vi "IPC-MQTT-Q driver.vi"(6 "Q Options":T2=enum."En Q N", 8 "error in (no error)":errorcluster, 9 "Message Data":variant, 10 "En Q":T1[](array[typedef]), 11 "Message":string) -> (0 "error out":errorcluster, 2 "Data":variant, 3 "State":string)   [LabVIEW 2020]
uses:
  Controls/IPC-MQTT-Q driver-Q Options.ctl
  Controls/IPC-MQTT-Q driver-En Q Element.ctl
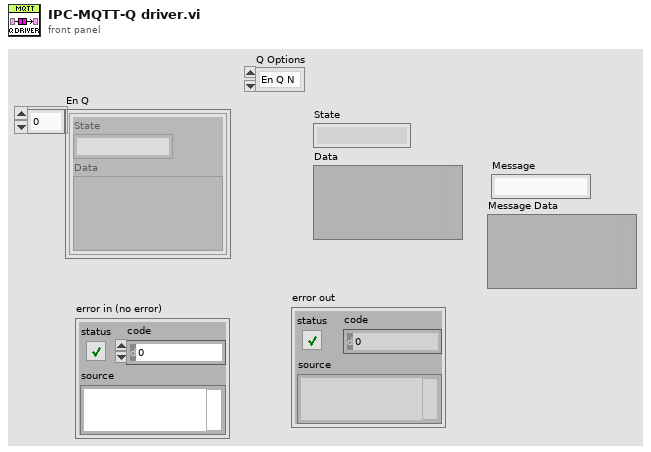
[diagram p1: front panel]
types:
  T1 = typedef "IPC-MQTT-Q driver-En Q Element.ctl" = cluster{"State":string, "Data":variant}
  T2 = typedef "IPC-MQTT-Q driver-Q Options.ctl" = enum16{"En Q", "En Q N", "De Q", "Init", "En Q N Stack", "Flush", "Close"}
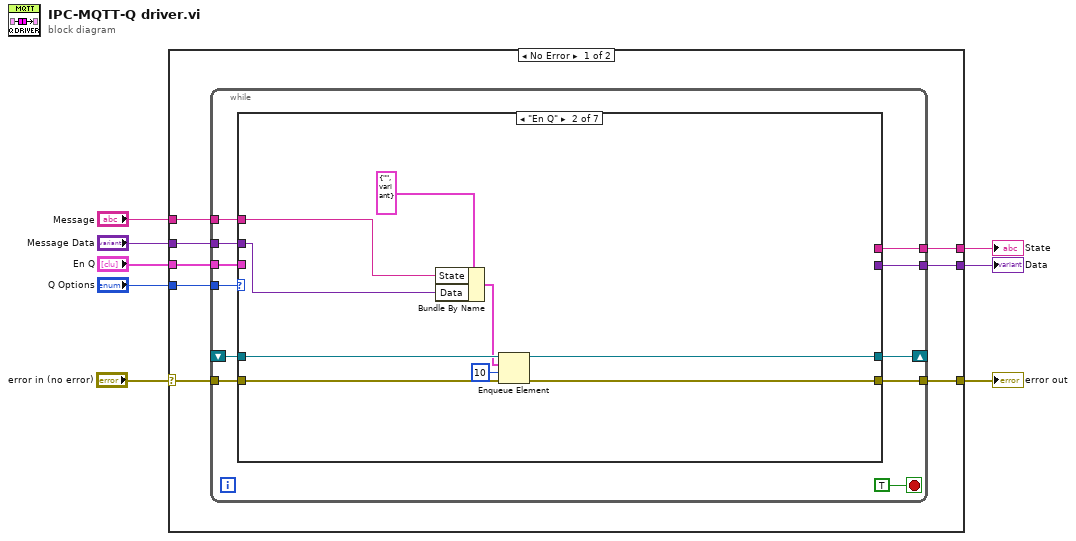
[diagram p0: block diagram]
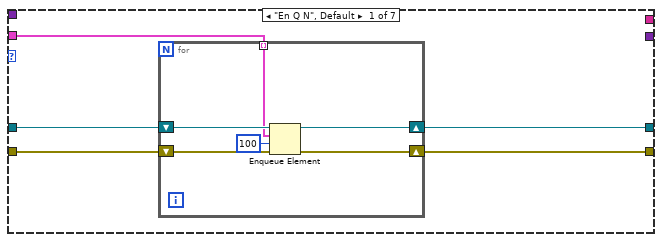
[diagram p2: hidden frame]
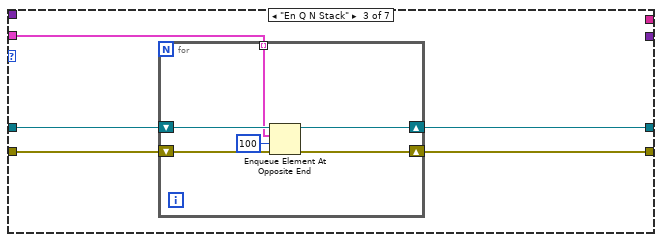
[diagram p3: hidden frame]
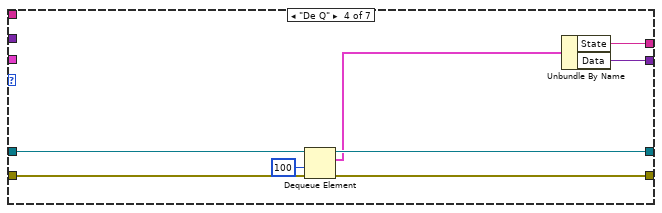
[diagram p4: hidden frame]
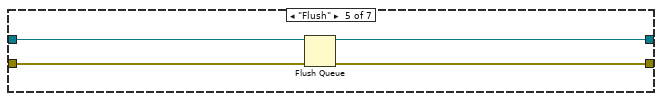
[diagram p5: hidden frame]
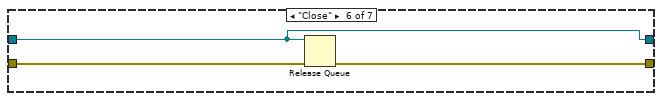
[diagram p6: hidden frame]
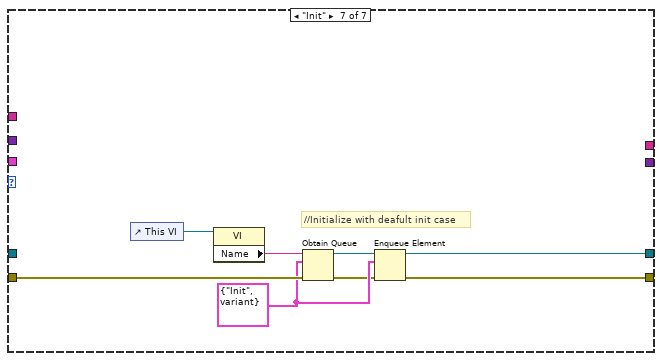
[diagram p7: hidden frame]
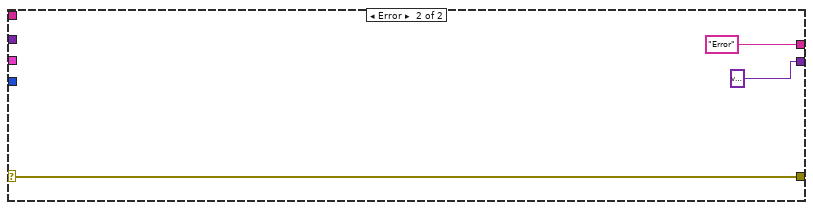
[diagram p8: hidden frame]
diagram:
  n1 = case shown="No Error" "error in (no error)" {
    selector: "error in (no error)" -> [w15 w83]
    tunnel: [w16 w83] -> w7
    tunnel: [w12 "Error"] -> w6
    tunnel: [w11 variant] -> w5
    tunnel: "Q Options" -> [w14 _]
    tunnel: "En Q" -> [w13 _]
    tunnel: "Message" -> [w10 _]
    tunnel: "Message Data" -> [w9 _]
    frame No Error {
      n2 = while {
        tunnel: [w25] -> w16
        tunnel: w15 -> [w26]
        tunnel: w14 -> [w24]
        tunnel: w13 -> [w23]
        shift-right: [w22] -> _
        shift-left: _ -> [w21]
        tunnel: [w20] -> w12
        tunnel: [w19] -> w11
        tunnel: w10 -> [w18]
        tunnel: w9 -> [w17]
        stop <- TRUE stop-if-true
        n3 = case shown="\"En Q\"" w24 {
          tunnel: w26 -> [w29 w44 w49 w64 w67 w72 w80]
          tunnel: [w30 w45 w50 w63 w68 w73 w74] -> w25
          tunnel: w23 -> [w28 _ w48 _ _ _ _]
          tunnel: [w31 w46 w51 w65 w69 w71 w77] -> w22
          tunnel: w21 -> [w32 w47 w52 w66 w70 w71 _]
          tunnel: [_ _ _ w60 _ _ _] -> w20
          tunnel: [_ _ _ w59 _ _ _] -> w19
          tunnel: w18 -> [_ w40 _ _ _ _ _]
          tunnel: w17 -> [_ w39 _ _ _ _ _]
          frame "En Q N", Default {
            n4 = for {
              shift-right: [w36] -> w30
              shift-left: w29 -> [w35]
              tunnel: w28 -> [w34] mode=indexing
              shift-right: [w37] -> w31
              shift-left: w32 -> [w38]
              n5 = Enqueue Element(queue=w38, element=w34, timeout in ms (-1)=100, error in (no error)=w35) -> (queue out=w37:refnum<queue>, error out=w36:errorcluster)  [unwired: 1 out]
            }
          }
          frame "En Q" {
            n6 = Bundle By Name(cluster=T1 {"State"="", "Data"=variant} ("En Q"), "State"=w40, "Data"=w39) -> (w41:T1)
            n7 = Enqueue Element(queue=w47, element=w41, timeout in ms (-1)=10, error in (no error)=w44) -> (queue out=w46:refnum<queue>, error out=w45:errorcluster)  [unwired: 1 out]
          }
          frame "En Q N Stack" {
            n8 = for {
              shift-right: [w56] -> w50
              shift-left: w49 -> [w55]
              tunnel: w48 -> [w54] mode=indexing
              shift-right: [w57] -> w51
              shift-left: w52 -> [w58]
              n9 = Enqueue Element At Opposite End(queue=w58, element=w54, timeout in ms (-1)=100, error in (no error)=w55) -> (queue out=w57:refnum<queue>, error out=w56:errorcluster)  [unwired: 1 out]
            }
          }
          frame "De Q" {
            n10 = Dequeue Element(queue=w66, timeout in ms (-1)=100, error in (no error)=w64) -> (queue out=w65:refnum<queue>, element=w61:T1, error out=w63:errorcluster)  [unwired: 1 out]
            n11 = Unbundle By Name(w61) -> ("State"=w60:string, "Data"=w59:variant)
          }
          frame "Flush" {
            n12 = Flush Queue(queue=w70, error in (no error)=w67) -> (queue out=w69:refnum<queue>, error out=w68:errorcluster)  [unwired: 1 out]
          }
          frame "Close" {
            n13 = Release Queue(queue=w71, error in (no error)=w72) -> (error out=w73:errorcluster)  [unwired: 1 in, 2 out]
          }
          frame "Init" {
            w76 = T1 {"State"="Init", "Data"=variant} ("En Q")
            # "//Initialize with deafult init case"
            n14 = control-ref of="This VI"() -> (w79:refnum<vi>)
            n15 = property class="VI"(reference=w79) -> ("Name"=w78:string)  [unwired: 1 in, 2 out]
            n16 = Obtain Queue(name (unnamed)=w78, element data type=w76, error in (no error)=w80) -> (queue out=w77:refnum<queue>, error out=w75:errorcluster)  [unwired: 2 in, 1 out]
            n17 = Enqueue Element(queue=w77, element=w76, error in (no error)=w75) -> (error out=w74:errorcluster)  [unwired: 1 in, 2 out]
          }
        }
      }
    }
    frame Error {
    }
  }
  "error out" <- w7
  "Data" <- w5
  "State" <- w6
